vi "CheckStatusLoop.vi"(1 "loop time":u32, 2 "StatusListRef":refnum<queue>, 3 "NotificationRef":refnum<notifier>, 4 "ListRef":refnum<queue>) -> ()   [LabVIEW 2012]
panel:
  out "错误输出":errorcluster
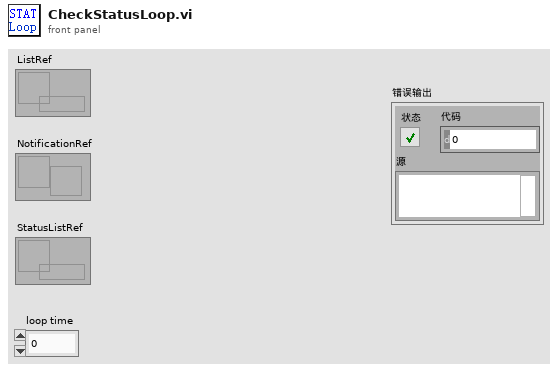
[diagram p1: front panel]
types:
  T1 = cluster{"output report":string, "output report":string, "output report":string, "output report":string, "output report":string}
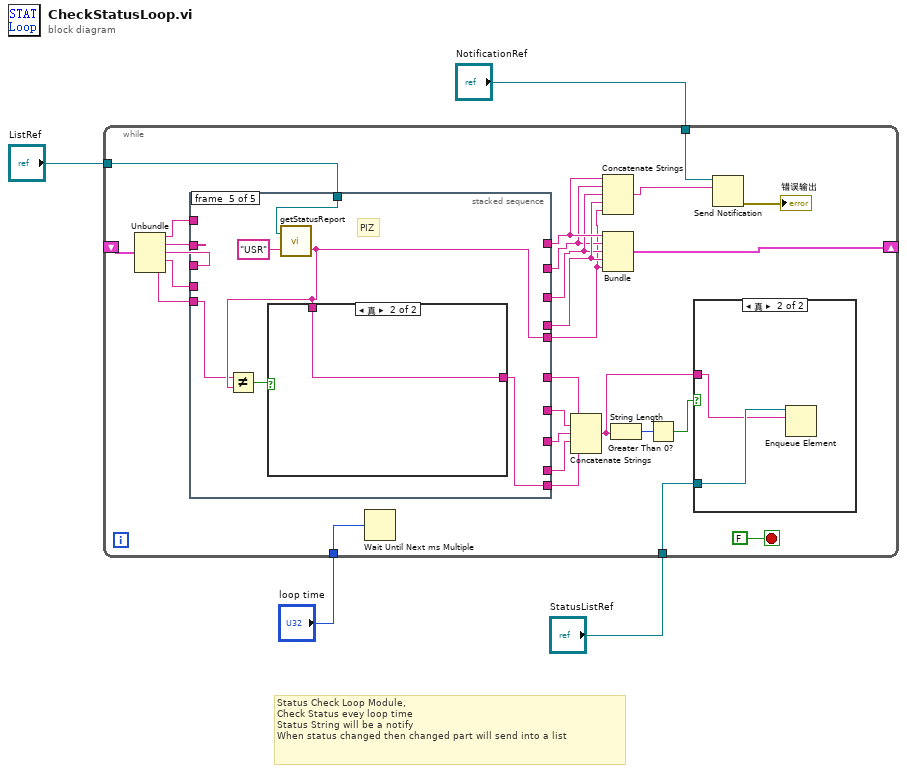
[diagram p0: block diagram]
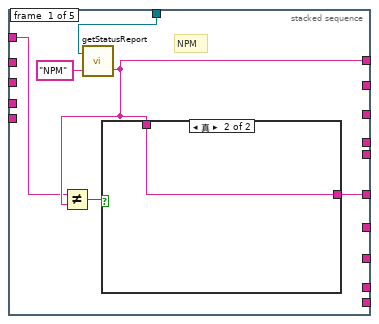
[diagram p3: hidden frame]
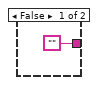
[diagram p4: hidden frame]
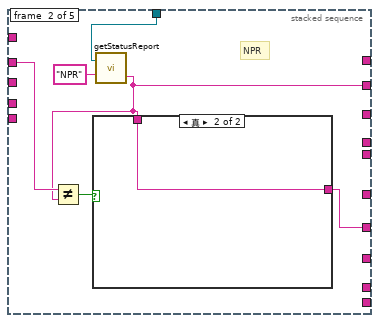
[diagram p5: hidden frame]
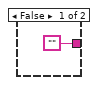
[diagram p6: hidden frame]
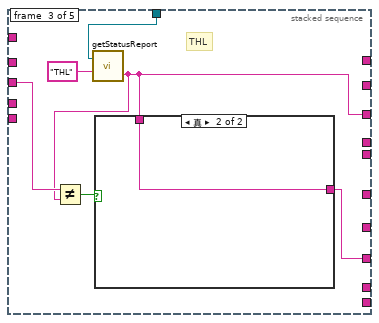
[diagram p7: hidden frame]
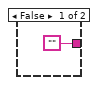
[diagram p8: hidden frame]
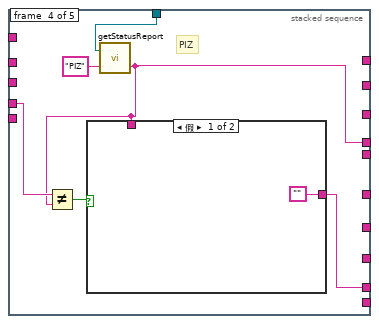
[diagram p9: hidden frame]
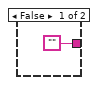
[diagram p11: hidden frame]
diagram:
  # "Status Check Loop Module,\nCheck Status evey loop time\nStatus String will be a notify\nWhen status changed then changed part will send into a list"
  n1 = while {
    tunnel: "ListRef" -> [w31]
    shift-right: [w29] -> _
    shift-left: _ -> [w28]
    tunnel: "loop time" -> [w23]
    tunnel: "NotificationRef" -> [w17]
    tunnel: "StatusListRef" -> [w9]
    stop <- FALSE stop-if-true
    n2 = Unbundle(w28) -> ("output report"=w27:string, "output report"=w25:string, "output report"=w26:string, "output report"=w24:string, "output report"=w7:string)
    n3 = stacked-sequence {
      tunnel: w31 -> [w39 w47 w55 w63 w71]
      tunnel: [w36 _ _ _ _] -> w16
      tunnel: [_ w43 _ _ _] -> w13
      tunnel: [_ _ w51 _ _] -> w14
      tunnel: [_ _ _ w58 _] -> w15
      tunnel: w27 -> [w35 _ _ _ _]
      tunnel: w26 -> [_ _ w53 _ _]
      tunnel: w25 -> [_ w44 _ _ _]
      tunnel: w24 -> [_ _ _ w60 _]
      tunnel: [_ _ _ w59 _] -> w21
      tunnel: [w34 _ _ _ _] -> w19
      tunnel: [_ _ w50 _ _] -> w22
      tunnel: [_ w42 _ _ _] -> w20
      tunnel: [_ _ _ _ w68] -> w6
      tunnel: [_ _ _ _ w67] -> w5
      tunnel: w7 -> [_ _ _ _ w66]
      frame #0 {
        # "NPM"
        n4 = call "getStatusReport.vi"("device"="NPM", "ListRef"=w39) -> ("output report"=w36:string)  [unwired: 1 in]
        n5 = Not Equal?(x=w35, y=w36) -> (x != y?=w37:bool)
        n6 = case shown="真" w37 {
          tunnel: ["" w41] -> w34
          tunnel: w36 -> [_ w41]
          frame False {
          }
          frame True {
          }
        }
      }
      frame #1 {
        # "NPR"
        n7 = call "getStatusReport.vi"("device"="NPR", "ListRef"=w47) -> ("output report"=w43:string)  [unwired: 1 in]
        n8 = Not Equal?(x=w44, y=w43) -> (x != y?=w45:bool)
        n9 = case shown="真" w45 {
          tunnel: ["" w49] -> w42
          tunnel: w43 -> [_ w49]
          frame False {
          }
          frame True {
          }
        }
      }
      frame #2 {
        # "THL"
        n10 = call "getStatusReport.vi"("device"="THL", "ListRef"=w55) -> ("output report"=w51:string)  [unwired: 1 in]
        n11 = Not Equal?(x=w53, y=w51) -> (x != y?=w52:bool)
        n12 = case shown="真" w52 {
          tunnel: ["" w57] -> w50
          tunnel: w51 -> [_ w57]
          frame False {
          }
          frame True {
          }
        }
      }
      frame #3 {
        # "PIZ"
        n13 = call "getStatusReport.vi"("device"="PIZ", "ListRef"=w63) -> ("output report"=w58:string)  [unwired: 1 in]
        n14 = Not Equal?(x=w60, y=w58) -> (x != y?=w61:bool)
        n15 = case shown="假" w61 {
          tunnel: ["" w65] -> w59
          tunnel: w58 -> [_ w65]
          frame False {
          }
          frame True {
          }
        }
      }
      frame #4 {
        # "PIZ"
        n16 = call "getStatusReport.vi"("device"="USR", "ListRef"=w71) -> ("output report"=w67:string)  [unwired: 1 in]
        n17 = Not Equal?(x=w66, y=w67) -> (x != y?=w69:bool)
        n18 = case shown="真" w69 {
          tunnel: ["" w73] -> w68
          tunnel: w67 -> [_ w73]
          frame False {
          }
          frame True {
          }
        }
      }
    }
    n19 = Wait Until Next ms Multiple(millisecond multiple=w23) -> ()  [unwired: 1 out]
    n20 = Concatenate Strings(w19, w20, w22, w21, w6) -> (w8:string)
    n21 = Concatenate Strings(w16, w13, w14, w15, w5) -> (w12:string)
    n22 = Bundle("output report"=w16, "output report"=w13, "output report"=w14, "output report"=w15, "output report"=w5) -> (w29:T1)  [unwired: 1 in]
    n23 = String Length(string=w8) -> (length=w18:i32)
    n24 = Greater Than 0?(x=w18) -> (x > 0?=w10:bool)
    n25 = case shown="真" w10 {
      tunnel: w9 -> [_ w33]
      tunnel: w8 -> [_ w32]
      frame False {
      }
      frame True {
        n26 = Enqueue Element(queue=w33, element=w32) -> ()  [unwired: 2 in, 3 out]
      }
    }
    n27 = Send Notification(notification=w12, notifier=w17) -> (error out=→"错误输出":errorcluster)  [unwired: 1 in, 1 out]
  }
